vi "Read To Char.vi"(6 "Char":string, 8 "error in (no error)":errorcluster, 11 "VisaComms in":refnum<class "VisaComms.lvclass">) -> (0 "error out":errorcluster, 2 "Response":string, 3 "VisaComms out":refnum<class "VisaComms.lvclass">)   [LabVIEW 2023, in "CTI.lvlib" / "VisaComms.lvclass"]
uses:
  VisaComms.lvclass
  VisaComms.lvclass/VisaComms.ctl
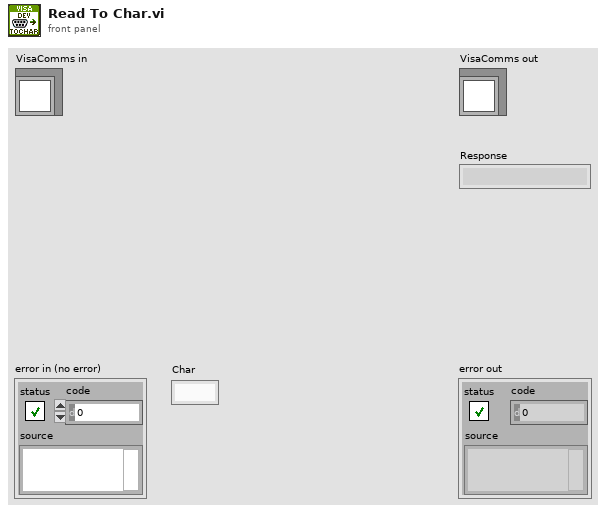
[diagram p1: front panel]
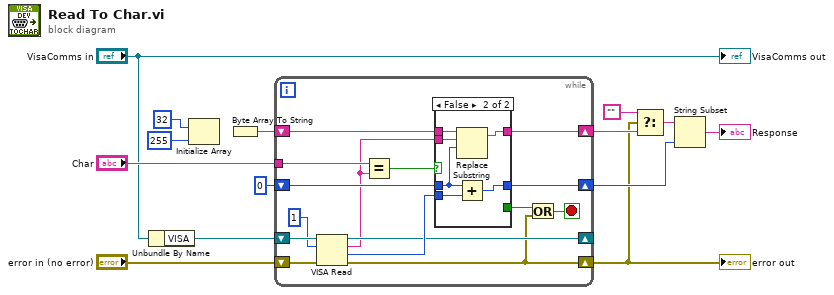
[diagram p0: block diagram]
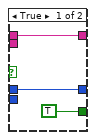
[diagram p2: hidden frame]
diagram:
  n1 = Unbundle By Name("VisaComms in") -> ("VISA"=w3:refnum<visa-resource-name>)
  n2 = Initialize Array(u8 32 ("element"), 255 ("dimension size")) -> ()  [unwired: 1 out]
  n3 = Byte Array To String() -> (string=w12:string)  [unwired: 1 in]
  n4 = while {
    shift-right: [w19] -> w1
    shift-left: "error in (no error)" -> [w28]
    shift-right: [w20] -> _
    shift-left: w3 -> [w29]
    shift-right: [w23] -> w11
    shift-left: w12 -> [w26]
    shift-right: [w24] -> w8
    shift-left: u32 0 -> [w25]
    tunnel: "Char" -> [w17]
    stop <- w21 stop-if-true
    n5 = VISA Read(VISA resource name=w29, byte count=u32 1, error in (no error)=w28) -> (VISA resource name out=w20:refnum<visa-resource-name>, read buffer=w15:string, return count=w22:u32, error out=w19:errorcluster)
    n6 = Equal?(x=w17, y=w15) -> (x = y?=w16:bool)
    n7 = case shown="False" w16 {
      tunnel: w26 -> [w32 w38]
      tunnel: w25 -> [w31 w37]
      tunnel: [w31 w36] -> w24
      tunnel: [w32 w35] -> w23
      tunnel: w22 -> [_ w34]
      tunnel: [TRUE _] -> w18
      tunnel: w15 -> [_ w33]
      frame True {
      }
      frame False {
        n8 = Replace Substring(3:w37, 4:w33, 5:w38) -> (1:w35:string)  [unwired: 1 in, 1 out]
        n9 = Add(x=w37, y=w34) -> (x+y=w36:u32)
      }
    }
    n10 = Or(x=w18, y=w19) -> (x .or. y?=w21:bool)
  }
  "error out" <- w1
  n11 = Select(t="", s=w1, f=w11) -> (s? t:f=w9:string)
  n12 = String Subset(string=w9, length (rest)=w8) -> (substring=→"Response":string)  [unwired: 1 in]
  "VisaComms out" <- "VisaComms in"
